vi "Main.vi"() -> ()   [LabVIEW 2019]
uses:
  Typedefs/#enum_State.ctl
  <vilib>/sound2/lvsound2.llb/Sound Data Format.ctl
  <vilib>/sound2/lvsound2.llb/Sampling Mode.ctl
  Typedefs/#cluster_ApplicationData.ctl
  <vilib>/sound2/lvsound2.llb/Sound File Refnum.ctl
  <vilib>/sound2/lvsound2.llb/Sound Input Task ID.ctl
  <vilib>/sound2/lvsound2.llb/Sound Input Read (DBL).vi
panel:
  out "Raw Data":waveform(dbl)[](graph)
  out "Spectrum Data":cluster{"f0":dbl, "df":dbl, "magnitude":dbl[]}[](graph)
  out "Threshold Exceeded?":bool
  in  "Threshold, dB":dbl=-100.0 format="%#_13g"
  in  "Upper Fc":dbl=3500.0 format="%#_13g"
  in  "Lower Fc":dbl=300.0 format="%#_13g"
  in  "Order":i32=6
  in  "Type":T1(ring)
  in  "Stop":bool
  # "FILTER SETTINGS"
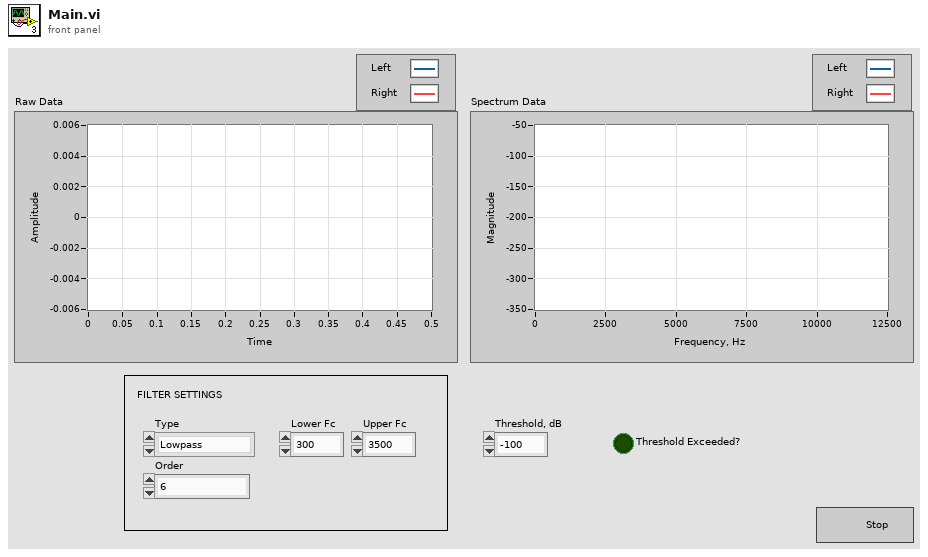
[diagram p1: front panel]
types:
  T1 = enum16{"Lowpass", "Highpass", "Bandpass", "Bandstop"}
  T2 = typedef "#enum_State.ctl" = enum16{"Init", "Acquisition", "Error Handler", "Exit"}
  T3 = typedef "Sound Data Format.ctl" = cluster{"sample rate (S/s)":dbl, "number of channels":i32, "bits per sample":i32}
  T4 = typedef "#cluster_ApplicationData.ctl" = cluster{"Sound file refnum":T5, "Acquisition task ID":T6, "Sound format":T3, "Number of samples/channel":i32}
  T5 = typedef "Sound File Refnum.ctl" = refnum<file>
  T6 = typedef "Sound Input Task ID.ctl" = u32
  T7 = typedef "Sampling Mode.ctl" = i32
  T8 = cluster{"Topology":enum16{"Off", "Butterworth", "Chebyshev", "Inverse Chebyshev", "Elliptic", "Bessel"}, "Type":enum16{"Lowpass", "Highpass", "Bandpass", "Bandstop"}, "Order":i32, "Lower Fc":dbl, "Upper Fc":dbl, "PB Ripple":dbl, "SB Attenuation":dbl}
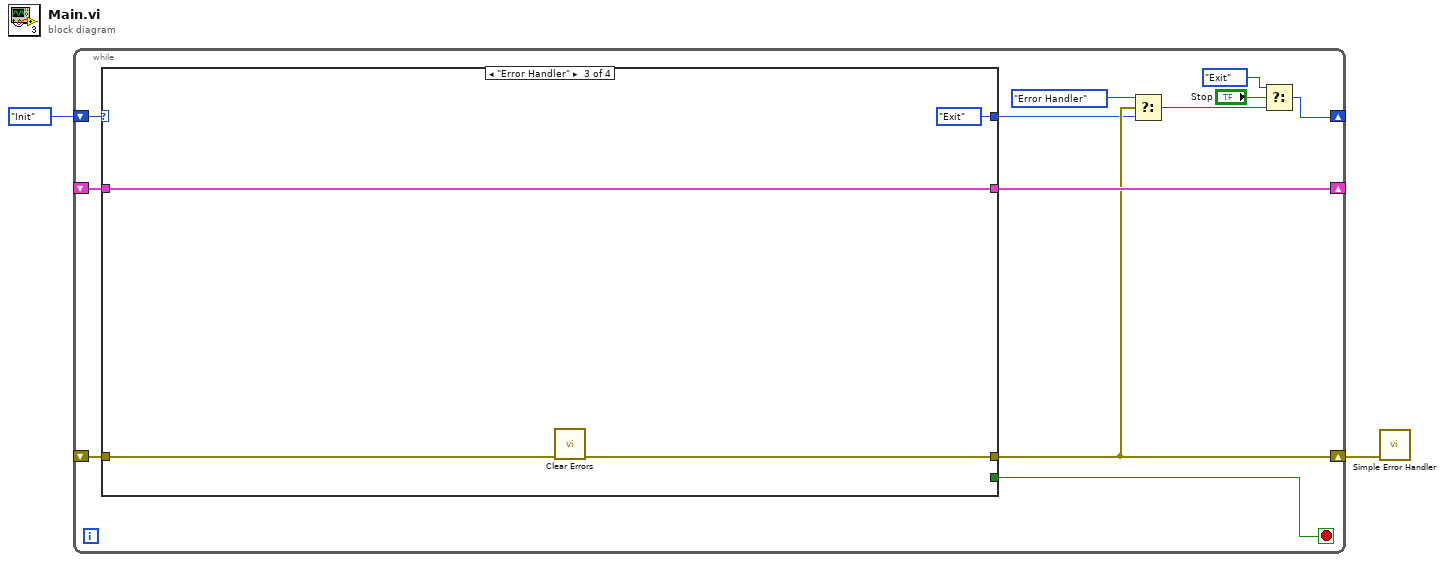
[diagram p0: block diagram]
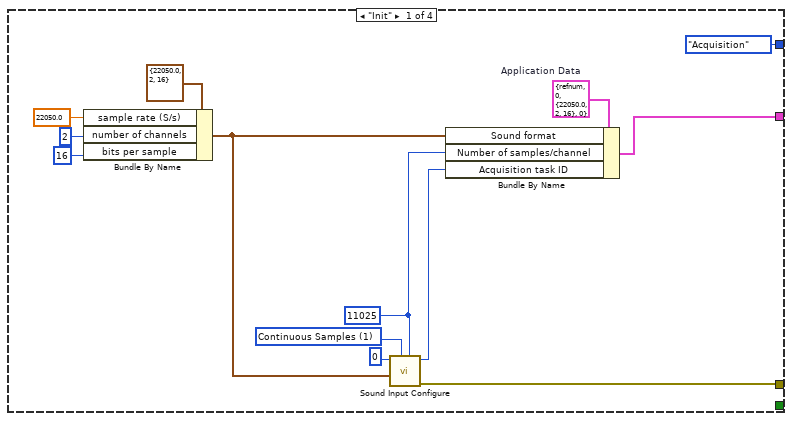
[diagram p2: hidden frame]
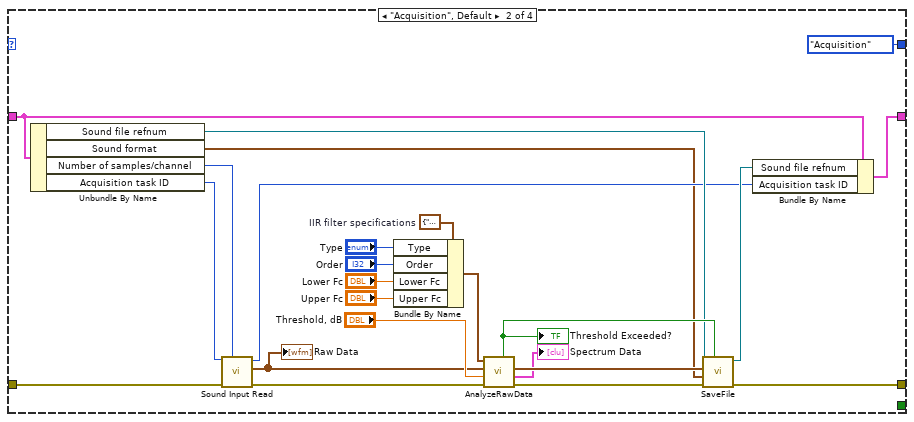
[diagram p3: hidden frame]
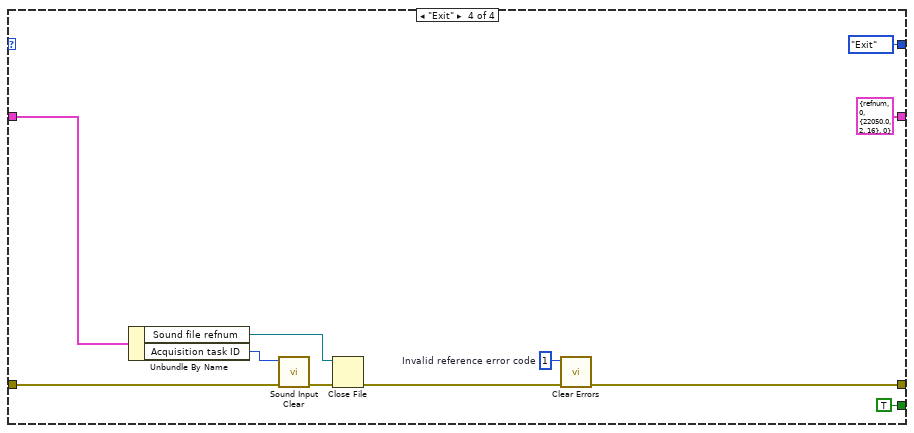
[diagram p4: hidden frame]
diagram:
  n1 = while {
    shift-right: [w5] -> _
    shift-left: #enum_State."Init" ("State") -> [w14]
    shift-right: [w12] -> _
    shift-left: _ -> [w13]
    shift-right: [w9] -> w2
    shift-left: _ -> [w11]
    stop <- w10 stop-if-true
    n2 = case shown="\"Error Handler\"" w14 {
      tunnel: w11 -> [_ w51 w55 w63]
      tunnel: [w19 w38 w53 w60] -> w9
      tunnel: w13 -> [_ w35 w54 w57]
      tunnel: [w20 w34 w54 T4 {"Sound file refnum"=refnum, "Acquisition task ID"=0, "Sound format"={"sample rate (S/s)"=22050.0, "number of channels"=2, "bits per sample"=16}, "Number of samples/channel"=0} ("Application Data")] -> w12
      tunnel: [#enum_State."Acquisition" ("State") #enum_State."Acquisition" ("State") #enum_State."Exit" ("State") #enum_State."Exit" ("State")] -> w6
      tunnel: [_ _ _ TRUE] -> w10
      frame "Init" {
        w21 = T4 {"Sound file refnum"=refnum, "Acquisition task ID"=0, "Sound format"={"sample rate (S/s)"=22050.0, "number of channels"=2, "bits per sample"=16}, "Number of samples/channel"=0}  # Application Data
        w16 = 11025 ("Number of Samples/ch")
        w27 = T7 1 items=["Finite Samples", "Continuous Samples"] ("sample mode")
        n3 = Bundle By Name(cluster=T3 {"sample rate (S/s)"=22050.0, "number of channels"=2, "bits per sample"=16} ("sound format"), "sample rate (S/s)"=22050.0 ("Sample rate (Hz)"), "number of channels"=2 ("#Channels"), "bits per sample"=16 ("Resolution (bits)")) -> (w18:T3)
        n4 = call <vilib>:"Sound Input Configure.vi"("number of samples/ch"=w16, "sample mode"=w27, "sound format"=w18, "device ID"=u32 0 ("Device")) -> ("error out"=w19:errorcluster, "task ID"=w17:T6)  [unwired: 6 in]
        n5 = Bundle By Name(cluster=w21, "Sound format"=w18, "Number of samples/channel"=w16, "Acquisition task ID"=w17) -> (w20:T4)
      }
      frame "Acquisition", Default {
        w50 = T8 {"Topology"=enum."Butterworth", "Type"=enum."Lowpass", "Order"=1, "Lower Fc"=100.0, "Upper Fc"=200.0, "PB Ripple"=1.0, "SB Attenuation"=60.0}  # IIR filter specifications
        n6 = Unbundle By Name(w35) -> ("Sound file refnum"=w36:T5, "Sound format"=w29:T3, "Number of samples/channel"=w30:i32, "Acquisition task ID"=w31:T6)
        n7 = call-poly <vilib>:"Sound Input Read.vi"("number of samples/ch"=w30, "error in (no error)"=w51, "task ID"=w31) -> ("error out"=w45:errorcluster, "data"=w43:waveform(dbl)[], "task ID out"=w32:T6)  [unwired: 6 in]
        "Raw Data" <- w43
        n8 = Bundle By Name(cluster=w50, "Type"="Type", "Order"="Order", "Lower Fc"="Lower Fc", "Upper Fc"="Upper Fc") -> (w42:T8)
        n9 = call "AnalyzeRawData.vi"("error in (no error)"=w45, "Threshold, dB"="Threshold, dB", "Raw Data"=w43, "IIR Filter Specifications"=w42) -> ("error out"=w39:errorcluster, "Power Spectrum / PSD"=→"Spectrum Data":cluster{"f0":dbl, "df":dbl, "magnitude":dbl[]}[], "Filtered Data"=w41:waveform(dbl)[], "Threshold Exceeded?"=w37:bool)  [unwired: 4 in]
        "Threshold Exceeded?" <- w37
        n10 = call "SaveFile.vi"("Threshold Exceeded?"=w37, "error in (no error)"=w39, "sound format"=w29, "Filtered Data"=w41, "sound file refnum in"=w36) -> ("error out"=w38:errorcluster, "sound file refnum out"=w33:T5)  [unwired: 5 in]
        n11 = Bundle By Name(cluster=w35, "Sound file refnum"=w33, "Acquisition task ID"=w32) -> (w34:T4)
      }
      frame "Error Handler" {
        n12 = call <vilib>:"Clear Errors.vi"("error in (no error)"=w55) -> ("error out"=w53:errorcluster)  [unwired: 5 in, 1 out]
      }
      frame "Exit" {
        w66 = 1  # Invalid reference error code
        n13 = Unbundle By Name(w57) -> ("Sound file refnum"=w61:T5, "Acquisition task ID"=w62:T6)
        n14 = call <vilib>:"Sound Input Clear.vi"("error in (no error)"=w63, "task ID"=w62) -> ("error out"=w64:errorcluster)  [unwired: 9 in]
        n15 = Close File(refnum=w61, error in=w64) -> (error out=w65:errorcluster)  [unwired: 1 out]
        n16 = call <vilib>:"Clear Errors.vi"("error in (no error)"=w65, "specific error code to clear (0: all)"=w66) -> ("error out"=w60:errorcluster)  [unwired: 4 in, 1 out]
      }
    }
    n17 = Select(t=#enum_State."Error Handler" ("State"), s=w9, f=w6) -> (s? t:f=w7:T2)
    n18 = Select(t=#enum_State."Exit" ("State"), s="Stop", f=w7) -> (s? t:f=w5:T2)
  }
  n19 = call <vilib>:"Simple Error Handler.vi"("error in (no error)"=w2) -> ()  [unwired: 4 in, 5 out]
